vi "Append XminiScan(MC).vi"(9 "Reference Data":T1={"Refrence data path"=path "", "Reference Rectangle"=[], "AOL Z"=0.0, "No of pixels in a miniscan "=[], "Threshold"=[], "No of miniscans"=[], "Full Frame Size"=0, "Reference Image"=refnum, "dwelltime"=0.1, "Zoom"=1.0, "Field of View"=0.0, "Z Step"=1, "Z pixels"=1, "Z Lines"=1, "Z Ignore"=1, "Laser"=1}, 11 "miniScan_Coordinates":T3) -> (3 "miniScan_Coordinates":T3)   [LabVIEW 2020]
uses:
  Typedefs/Reference_Globals.ctl
  <vilib>/vision/Image Controls.llb/IMAQ Image.ctl
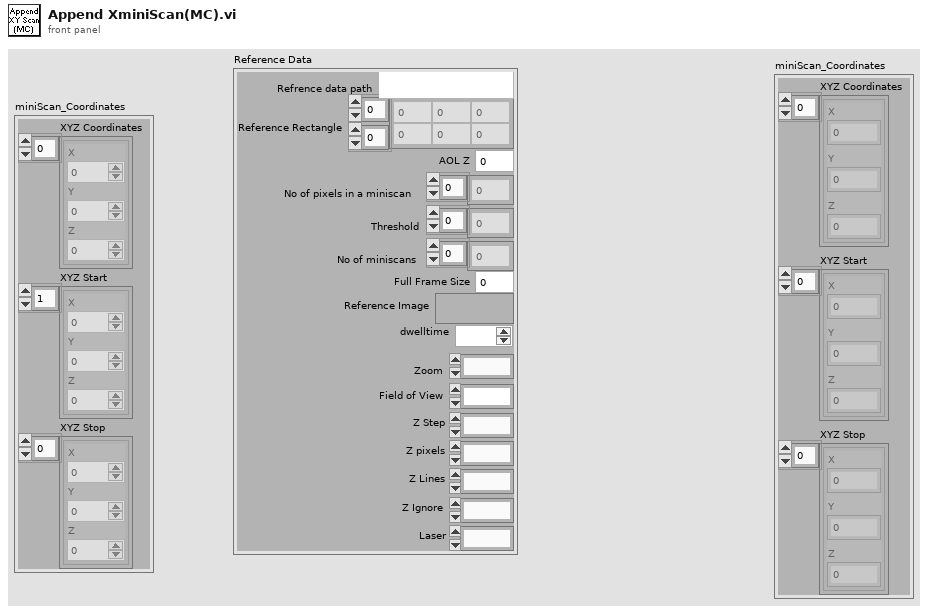
[diagram p1: front panel]
types:
  T1 = typedef "Reference_Globals.ctl" = cluster{"Refrence data path":path, "Reference Rectangle":i16[][], "AOL Z":dbl, "No of pixels in a miniscan ":i32[], "Threshold":i16[], "No of miniscans":i32[], "Full Frame Size":u16, "Reference Image":T2, "dwelltime":dbl, "Zoom":dbl, "Field of View":dbl, "Z Step":i8, "Z pixels":i32, "Z Lines":u8, "Z Ignore":u8, "Laser":u8}
  T2 = typedef "IMAQ Image.ctl" = refnum<image>
  T3 = cluster{"XYZ Coordinates":cluster{"X":sgl, "Y":sgl, "Z":sgl}[], "XYZ Start":cluster{"X":dbl, "Y":dbl, "Z":dbl}[], "XYZ Stop":cluster{"X":dbl, "Y":dbl, "Z":dbl}[]}
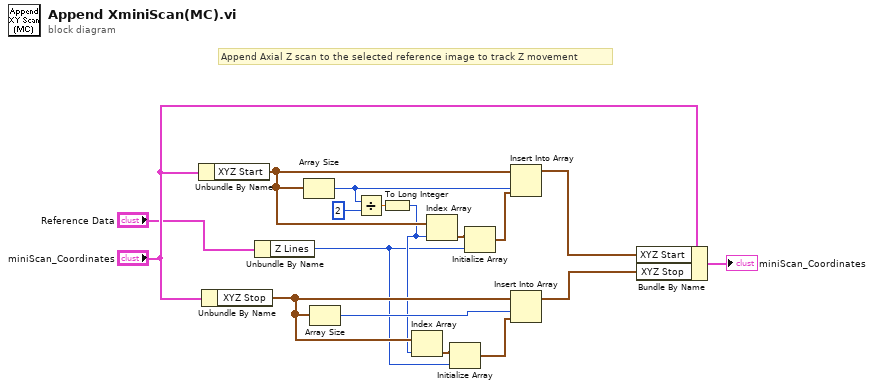
[diagram p0: block diagram]
diagram:
  # "Append Axial Z scan to the selected reference image to track Z movement"
  n1 = Unbundle By Name("miniScan_Coordinates") -> ("XYZ Start"=w12:cluster{"X":dbl, "Y":dbl, "Z":dbl}[])
  n2 = Unbundle By Name("miniScan_Coordinates") -> ("XYZ Stop"=w4:cluster{"X":dbl, "Y":dbl, "Z":dbl}[])
  n3 = Unbundle By Name("Reference Data") -> ("Z Lines"=w1:u8)
  n4 = Array Size(array=w12) -> (size(s)=w11:i32)
  n5 = Array Size(array=w4) -> (size(s)=w13:i32)
  n6 = Divide(x=w11, y=i16 2) -> (x/y=w9:dbl)
  n7 = To Long Integer(number=w9) -> (32bit integer=w3:i32)
  n8 = Index Array(array=w4, index=w3) -> (element=w5:cluster{"X":dbl, "Y":dbl, "Z":dbl})
  n9 = Index Array(array=w12, index=w3) -> (element=w8:cluster{"X":dbl, "Y":dbl, "Z":dbl})
  n10 = Initialize Array(w5, w1) -> (w2:cluster{"X":dbl, "Y":dbl, "Z":dbl}[])
  n11 = Initialize Array(w8, w1) -> (w6:cluster{"X":dbl, "Y":dbl, "Z":dbl}[])
  n12 = Insert Into Array(array=w12, index=w11, new element=w6) -> (w16:cluster{"X":dbl, "Y":dbl, "Z":dbl}[])
  n13 = Insert Into Array(array=w4, index=w13, new element=w2) -> (w15:cluster{"X":dbl, "Y":dbl, "Z":dbl}[])
  n14 = Bundle By Name(cluster="miniScan_Coordinates", "XYZ Start"=w16, "XYZ Stop"=w15) -> (→"miniScan_Coordinates":T3)
